vi "SIGNAL GENERATOR.vi"() -> ()   [LabVIEW 2018]
uses:
  <vilib>/measure/NI_MABase.lvlib
panel:
  in  "stop 2":bool
  out "STRIP Chart":dbl(graph)
  out "SWEEP CHART":dbl(graph)
  out "SCOPE Chart":dbl(graph)
  in  "signal type":T1(ring)
  in  "amplitude":dbl=1.0 format="%0.2p"
  in  "frequency":dbl=10.0 format="%0.2p"
  in  "stop":bool
  out "Waveform Graph":waveform(dbl)(graph)
  out "STRIP Chart":dbl(graph)
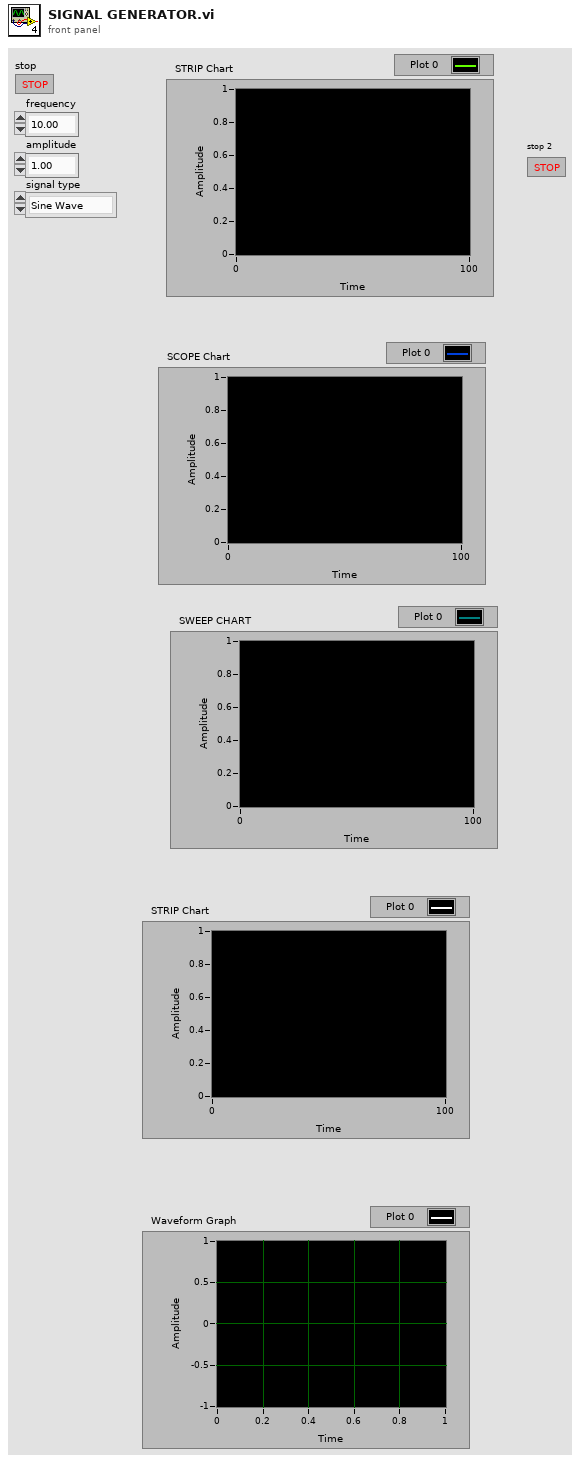
[diagram p1: front panel]
types:
  T1 = enum16{"Sine Wave", "Triangle Wave", "Square Wave", "Sawtooth Wave"}
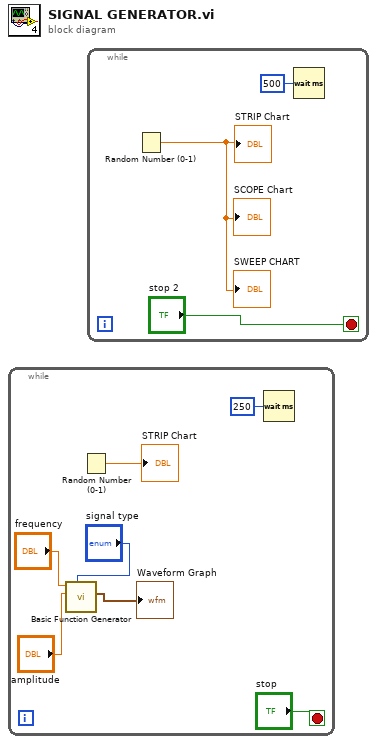
[diagram p0: block diagram]
diagram:
  n1 = while {
    stop <- "stop" stop-if-true
    n2 = call <vilib>:"Basic Function Generator.vi"("signal type"="signal type", "amplitude"="amplitude", "frequency"="frequency") -> ("signal out"=→"Waveform Graph":waveform(dbl))  [unwired: 6 in, 2 out]
    n3 = Random Number (0-1)() -> (number: 0 to 1=→"STRIP Chart":dbl)
    n4 = Wait (ms)(milliseconds to wait=u32 250) -> ()  [unwired: 1 out]
  }
  n5 = while {
    stop <- "stop 2" stop-if-true
    n6 = Random Number (0-1)() -> (number: 0 to 1=→"SWEEP CHART" →"SCOPE Chart" →"STRIP Chart":dbl)
    n7 = Wait (ms)(milliseconds to wait=u32 500) -> ()  [unwired: 1 out]
  }
